vi "isBlack.vi"(1 "BlackBOND":dbl) -> (0 "isBlack":bool)   [LabVIEW 2013]
uses:
  <vilib>/NXT/Block Support/NXT_InputPort.ctl
  <vilib>/NXT/Dual Mode Library/Sensors/EV3_Color_Reflect.vi
panel:
  out "Scaled Value":sgl
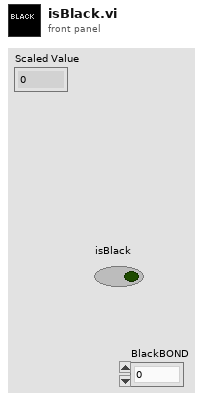
[diagram p1: front panel]
types:
  T1 = typedef "NXT_InputPort.ctl" = u32
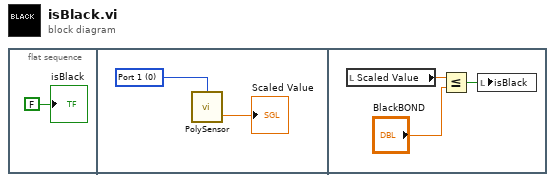
[diagram p0: block diagram]
diagram:
  n1 = flat-sequence {
    frame #0 {
      "isBlack" <- FALSE ("Boolean")
    }
    frame #1 {
      w2 = T1 0 items=["Port 1", "Port 2", "Port 3", "Port 4"] ("Port (Port 1)")
      n2 = call-poly <vilib>:"PolySensor.vi"("Port (Port 1)"=w2) -> ("Scaled Value"=→"Scaled Value":sgl)  [unwired: 2 in, 1 out]
    }
    frame #2 {
      n3 = local read "Scaled Value"() -> (w6:sgl)
      n4 = Less Or Equal?(x=w6, y="BlackBOND") -> (x <= y?=w5:bool)
      n5 = local write "isBlack"(w5) -> ()
    }
  }
